vi "WRP Wait For Region Ready.vi"(8 "error in (no error)":errorcluster, 11 "timeout_ms":i32) -> (0 "error out":errorcluster, 3 "function return":i32)   [LabVIEW 2018, in "SesWrapper.lvlib"]
doc: "int STDCALL WRP_WaitForRegionReady(int timeout_ms);"
uses:
  SesWrapper.lvlib
  build/Debug/SESWrapper.dll
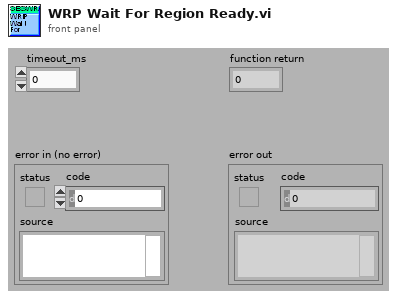
[diagram p1: front panel]
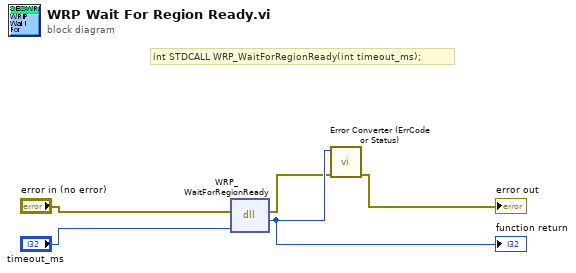
[diagram p0: block diagram]
diagram:
  # "int STDCALL WRP_WaitForRegionReady(int timeout_ms);"
  n1 = dll-call lib="C:/Development/svn/seswrapper-lib/build/Debug/SESWrapper.*" fn="WRP_WaitForRegionReady"(error in="error in (no error)", "timeout_ms"="timeout_ms") -> (error out=w2:errorcluster, w5:i32)  [unwired: 3 in, 1 out]
  "function return" <- w5
  n2 = call "Error Converter (ErrCode or Status).vi"("error in (no error)"=w2, "error code"=w5) -> ("error out"=→"error out":errorcluster)  [unwired: 9 in]
